vi "Init XML handler.vi"(8 "error in (no error)":errorcluster, 10 "Output File Folder":path, 11 "Test Framework in":refnum<class "Test Framework.lvclass">) -> (0 "error out":errorcluster, 3 "Test Framework out":refnum<class "Test Framework.lvclass">)   [LabVIEW 2020, in "Test Framework.lvclass"]
uses:
  Test Framework.lvclass
  XML Handler/XML Handler.lvclass
  Test Framework.lvclass/Test Framework.ctl
  Devices/Device.lvclass
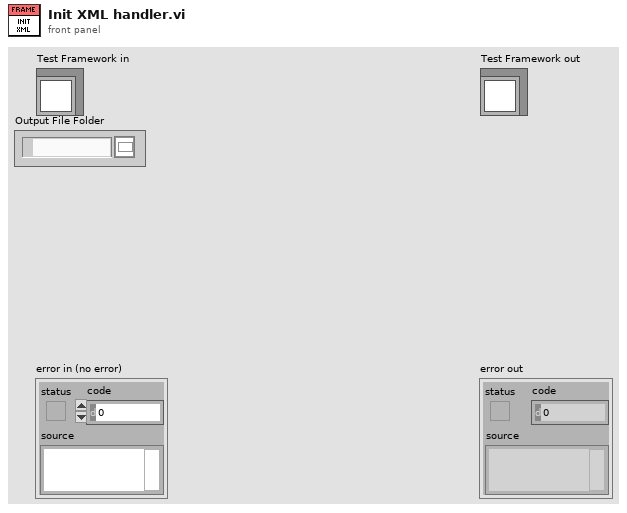
[diagram p1: front panel]
types:
  T1 = typedef "Device.lvclass/Device Information Cluster.ctl" = cluster{"Device Info":string[][], "Default Values":T2[], "Fetched info":string[][]}
  T2 = typedef "PIC-Device.lvclass/Register to Write.ctl" = cluster{"Register":u32, "Value":u32, "Dev Address":u32, "Physical Adress":u32}
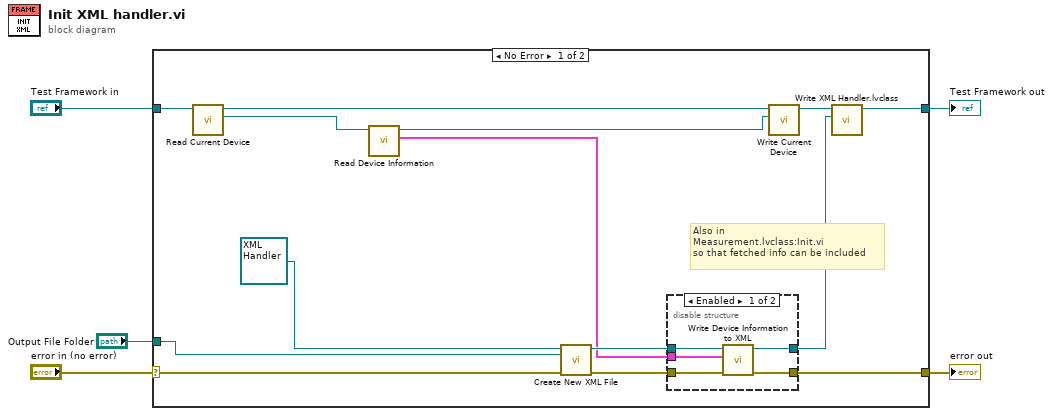
[diagram p0: block diagram]
diagram:
  n1 = case shown="No Error" "error in (no error)" {
    selector: "error in (no error)" -> [w6 w28]
    tunnel: [w9 w28] -> w4
    tunnel: [w11 w27] -> w2
    tunnel: "Test Framework in" -> [w15 w27]
    tunnel: "Output File Folder" -> [w18 _]
    frame No Error {
      # "Also in \nMeasurement.lvclass:Init.vi\nso that fetched info can be included"
      n2 = call-dynamic "Read Current Device.vi"("Test Framework in"=w15) -> ("Current Device.lvclass"=w7:refnum<class "Device.lvclass">, "Test Framework out"=w14:refnum<class "Test Framework.lvclass">)  [unwired: 9 in]
      n3 = call-dynamic "Read Device Information.vi"("Device in"=w7) -> ("Device Info"=w8:T1[], "Device out"=w13:refnum<class "Device.lvclass">)  [unwired: 8 in, 1 out]
      n4 = call "Create New XML File.vi"("error in (no error)"=w6, "Output File Folder"=w18, "XML Handler in"=refnum<class "XML Handler.lvclass"> refnum ("XML Handler.lvclass")) -> ("error out"=w16:errorcluster, "XML Handler out"=w17:refnum<class "XML Handler.lvclass">)  [unwired: 7 in]
      n5 = disable-structure shown="Enabled" {
        disable-tunnel: w17 -> [w24 w25]
        disable-tunnel: w16 -> [w23 w26]
        disable-tunnel: [w22 w25] -> w10
        disable-tunnel: [w21 w26] -> w9
        disable-tunnel: w8 -> [w20 _]
        frame Enabled {
          n6 = call "Write Device Information to XML.vi"("error in (no error)"=w23, "Device Information"=w20, "XML Handler in"=w24) -> ("error out"=w21:errorcluster, "XML Handler out"=w22:refnum<class "XML Handler.lvclass">)  [unwired: 7 in]
        }
        frame Disabled {
        }
      }
      n7 = call-dynamic "Write Current Device.vi"("Current Device.lvclass"=w13, "Test Framework in"=w14) -> ("Test Framework out"=w12:refnum<class "Test Framework.lvclass">)  [unwired: 9 in]
      n8 = call "Write XML Handler.lvclass.vi"("XML Handler.lvclass"=w10, "Test Framework in"=w12) -> ("Test Framework out"=w11:refnum<class "Test Framework.lvclass">)  [unwired: 9 in]
    }
    frame Error {
    }
  }
  "error out" <- w4
  "Test Framework out" <- w2
